vi "refresh group data.vi"(8 "error in":errorcluster, 9 "specification":T1[](array[typedef]), 10 "group in":T3, 11 "data table in":T3) -> (0 "error out":errorcluster, 2 "group out":T3, 3 "data table out":T3)   [LabVIEW 2013, in "data bus values.lvlib"]
doc: "Accepts a primary data table and a subgroup data table, and copies data from the main table into the group."
uses:
  data bus values.lvlib
  data table.ctl
  group specification.ctl
  tag/Data Type.ctl
  data polymorphs/read many/read Doubles.vi
  data polymorphs/write all/write all Doubles.vi
  data polymorphs/read many/read I64s.vi
  data polymorphs/write all/write all I64s.vi
  data polymorphs/read many/read Booleans.vi
  data polymorphs/write all/write all Booleans.vi
  data polymorphs/read many/read Array of Doubles.vi
  data polymorphs/write all/write all Array of Doubles.vi
  data polymorphs/read many/read Array of I64s.vi
  data polymorphs/write all/write all Array of I64s.vi
  data polymorphs/read many/read Variants.vi
  data polymorphs/write all/write all Variants.vi
  data bus error generator.vi
  tag/data bus tag description.lvclass
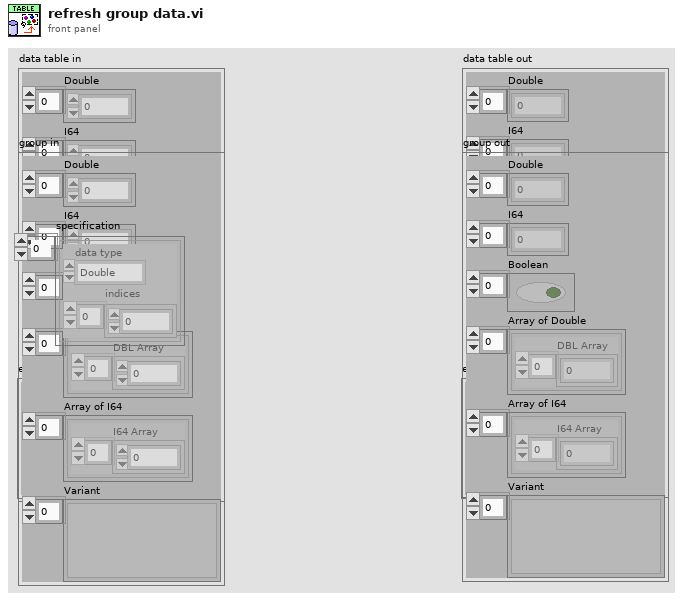
[diagram p1: front panel]
types:
  T1 = typedef "data bus values.lvlib/group specification.ctl" = cluster{"data type":T2, "indices":i32[]}
  T2 = typedef "data bus tag description.lvclass/Data Type.ctl" = enum16{"Double", "I64", "Boolean", "Array of Double", "Array of I64", "Variant"}
  T3 = typedef "data bus values.lvlib/data table.ctl" = cluster{"Double":dbl[], "I64":i64[], "Boolean":bool[], "Array of Double":cluster{"DBL Array":dbl[]}[], "Array of I64":cluster{"I64 Array":i64[]}[], "Variant":variant[]}
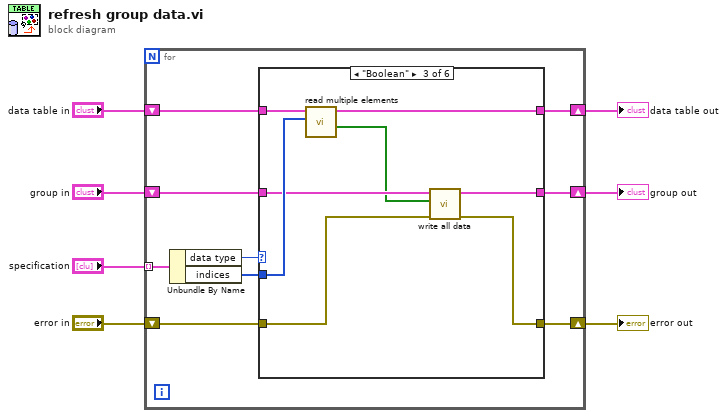
[diagram p0: block diagram]
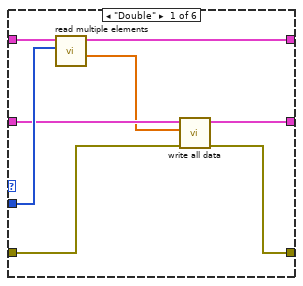
[diagram p2: hidden frame]
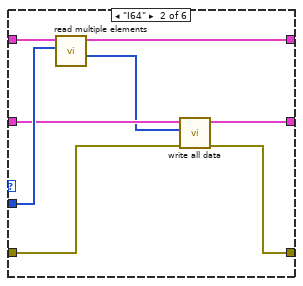
[diagram p3: hidden frame]
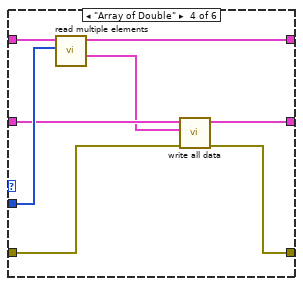
[diagram p4: hidden frame]
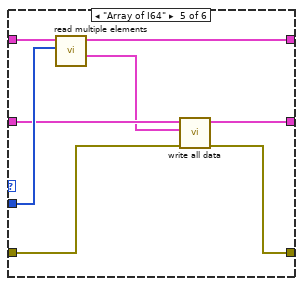
[diagram p5: hidden frame]
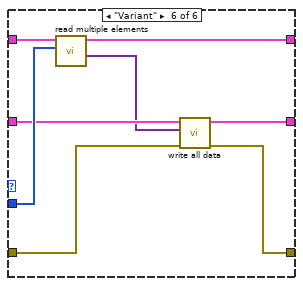
[diagram p6: hidden frame]
diagram:
  n1 = for {
    shift-right: [w11] -> w4
    shift-left: "error in" -> [w10]
    shift-right: [w12] -> w5
    shift-left: "data table in" -> [w13]
    shift-right: [w8] -> w2
    shift-left: "group in" -> [w9]
    tunnel: "specification" -> [w16] mode=indexing
    n2 = Unbundle By Name(w16) -> ("data type"=w15:T2, "indices"=w14:i32[])
    n3 = case shown="\"Boolean\"" w15 {
      tunnel: w14 -> [w22 w30 w38 w46 w54 w62]
      tunnel: w13 -> [w24 w32 w40 w48 w56 w64]
      tunnel: [w23 w31 w39 w47 w55 w63] -> w12
      tunnel: [w19 w27 w35 w43 w51 w59] -> w11
      tunnel: w10 -> [w20 w28 w36 w44 w52 w60]
      tunnel: w9 -> [w21 w29 w37 w45 w53 w61]
      tunnel: [w18 w26 w34 w42 w50 w58] -> w8
      frame "Double" {
        n4 = call-poly "read multiple elements.vi"("indices"=w22, "data table in"=w24) -> ("values"=w17:dbl[], "data table out"=w23:T3)  [unwired: 8 in]
        n5 = call-poly "write all data.vi"("error in"=w20, "values"=w17, "data table in"=w21) -> ("error out"=w19:errorcluster, "data table out"=w18:T3)  [unwired: 7 in]
      }
      frame "I64" {
        n6 = call-poly "read multiple elements.vi"("indices"=w30, "data table in"=w32) -> ("values"=w25:i64[], "data table out"=w31:T3)  [unwired: 8 in]
        n7 = call-poly "write all data.vi"("error in"=w28, "values"=w25, "data table in"=w29) -> ("error out"=w27:errorcluster, "data table out"=w26:T3)  [unwired: 7 in]
      }
      frame "Boolean" {
        n8 = call-poly "read multiple elements.vi"("indices"=w38, "data table in"=w40) -> ("values"=w33:bool[], "data table out"=w39:T3)  [unwired: 8 in]
        n9 = call-poly "write all data.vi"("error in"=w36, "values"=w33, "data table in"=w37) -> ("error out"=w35:errorcluster, "data table out"=w34:T3)  [unwired: 7 in]
      }
      frame "Array of Double" {
        n10 = call-poly "read multiple elements.vi"("indices"=w46, "data table in"=w48) -> ("values"=w41:cluster{"Array":dbl[]}[], "data table out"=w47:T3)  [unwired: 8 in]
        n11 = call-poly "write all data.vi"("error in"=w44, "values"=w41, "data table in"=w45) -> ("error out"=w43:errorcluster, "data table out"=w42:T3)  [unwired: 7 in]
      }
      frame "Array of I64" {
        n12 = call-poly "read multiple elements.vi"("indices"=w54, "data table in"=w56) -> ("values"=w49:cluster{"Array":i64[]}[], "data table out"=w55:T3)  [unwired: 8 in]
        n13 = call-poly "write all data.vi"("error in"=w52, "values"=w49, "data table in"=w53) -> ("error out"=w51:errorcluster, "data table out"=w50:T3)  [unwired: 7 in]
      }
      frame "Variant" {
        n14 = call-poly "read multiple elements.vi"("indices"=w62, "data table in"=w64) -> ("values"=w57:variant[], "data table out"=w63:T3)  [unwired: 8 in]
        n15 = call-poly "write all data.vi"("error in"=w60, "values"=w57, "data table in"=w61) -> ("error out"=w59:errorcluster, "data table out"=w58:T3)  [unwired: 7 in]
      }
    }
  }
  "error out" <- w4
  "data table out" <- w5
  "group out" <- w2
